vi "t2point.vi"(1 "t/point":T1(ring)) -> (0 "ps/point":u32)   [LabVIEW 2011]
panel:
  # "=>"
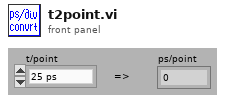
[diagram p1: front panel]
types:
  T1 = enum16{"25 ps", "50 ps", "100 ps", "200 ps", "400 ps", "800 ps", "2 ns"}
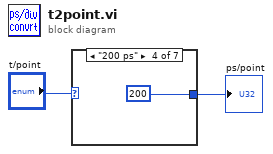
[diagram p0: block diagram]
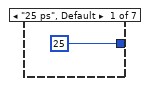
[diagram p2: hidden frame]
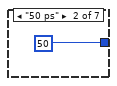
[diagram p3: hidden frame]
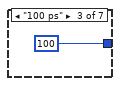
[diagram p4: hidden frame]
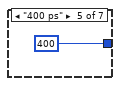
[diagram p5: hidden frame]
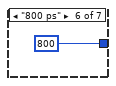
[diagram p6: hidden frame]
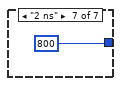
[diagram p7: hidden frame]
diagram:
  n1 = case shown="\"200 ps\"" "t/point" {
    tunnel: [25 50 100 200 400 800 800] -> w2
    frame "25 ps", Default {
    }
    frame "50 ps" {
    }
    frame "100 ps" {
    }
    frame "200 ps" {
    }
    frame "400 ps" {
    }
    frame "800 ps" {
    }
    frame "2 ns" {
    }
  }
  "ps/point" <- w2
